vi "Close.vi"(8 "ErrorIn":errorcluster, 11 "OpenCVCamIn":refnum<class "OpenCVCam.lvclass">) -> (0 "ErrorOut":errorcluster, 3 "OpenCVCamOut":refnum<class "OpenCVCam.lvclass">)   [LabVIEW 2021, in "OpenCVCam.lvclass"]
uses:
  OpenCVCam.lvclass
  C:/Localdata/Projects/TriekselSoft/TriekselsoftApplicationFramework/Source/.Externals/Library_YAF/YActor/YActor.lvclass
  .Externals/Library_YAF/YActor/YActor.lvclass/YActor.ctl
  .Externals/Library_YAF/YActor/ExeCmd_sync.vi
  .Externals/Library_YAF/YActor/private/SendCommand.vi
  .Externals/Library_YAF/YActor/private/WaitForReply.vi
  .Externals/Library_YAF/YActor/private/CreateLocalVI.vi
  .Externals/Library_YAF/YActor/private/ExeuteInlineVI.vi
  .Externals/Library_YAF/YActor/private/GetRemoteVIRef.vi
  .Externals/Library_YAF/YActor/private/GetNameOfVI.vi
  .Externals/Library_YAF/YActor/QuickCast.vi
  .Externals/Library_YAF/YActor/private/VINameProperty.vi
  .Externals/Library_YAF/YActor/private/MessageCounter.vi
  .Externals/Library_YAF/YActor/InlineReferencePool.vi
  .Externals/Library_YAF/YActor/private/ExecuteVI.vi
  .Externals/Library_YAF/YActor/YActor.lvclass
  C:/Localdata/Projects/TriekselSoft/TriekselsoftApplicationFramework/Source/.Externals/Library_YAF/YAFTAF/YAFTAF.lvclass
  C:/Localdata/Projects/TriekselSoft/TriekselsoftApplicationFramework/Source/.Externals/Interface_UserInterface_IFrontPanel/IFrontPanel/IFrontPanel.lvclass
  C:/Localdata/Projects/TriekselSoft/TriekselsoftApplicationFramework/Source/IInterface/IInterface.lvclass
  C:/Localdata/Projects/TriekselSoft/TriekselsoftApplicationFramework/Source/.Externals/Interface_Object_ICreateDestroy/ICreateDestroy/ICreateDestroy.lvclass
  C:/Localdata/Projects/TriekselSoft/TriekselsoftApplicationFramework/Source/.Externals/Interface_Object_IPersistentData/IPersistentData/IPersistentData.lvclass
  C:/Localdata/Projects/TriekselSoft/TriekselsoftApplicationFramework/Source/.Externals/Interface_TAF_ITAFObject/ITAFObject/ITAFObject.lvclass
  C:/Localdata/Projects/TriekselSoft/TriekselsoftApplicationFramework/Source/YAFTAFObjects/OpenCVCam/OpenCVCam.lvclass
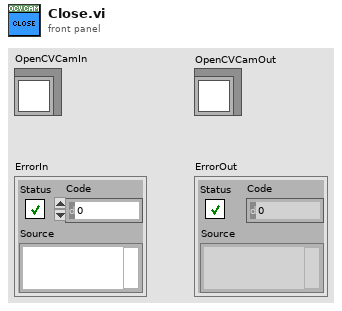
[diagram p1: front panel]
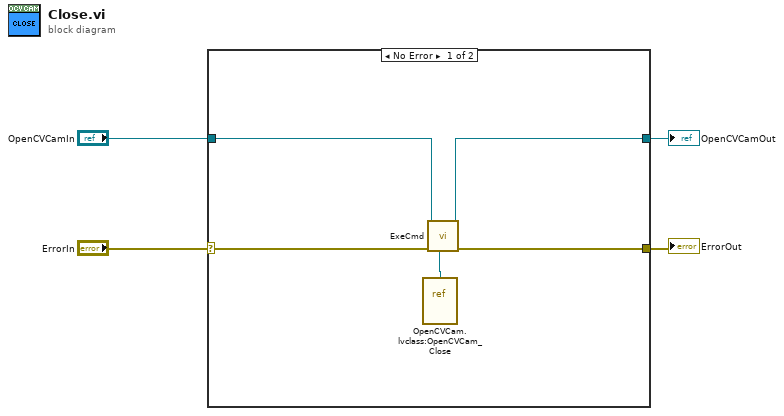
[diagram p0: block diagram]
diagram:
  n1 = case shown="No Error" "ErrorIn" {
    selector: "ErrorIn" -> [w9 w11]
    tunnel: [w8 w11] -> w3
    tunnel: [w5 w10] -> w1
    tunnel: "OpenCVCamIn" -> [w6 w10]
    frame No Error {
      n2 = vi-ref "OpenCVCam.lvclass:OpenCVCam_Close.vi"() -> (w7:refnum<vi>)
      n3 = call-poly "ExeCmd.vi"("CmdVIRef"=w7, "ErrorIn"=w9, "YActorIn"=w6) -> ("ErrorOut"=w8:errorcluster, "YActorOut"=w5:refnum<class "OpenCVCam.lvclass">)  [unwired: 6 in, 1 out]
    }
    frame Error {
    }
  }
  "ErrorOut" <- w3
  "OpenCVCamOut" <- w1
